vi "Vission Assistant.vi"() -> ()   [LabVIEW 2018]
uses:
  <vilib>/Rock Robotics/Network Tables/NT Read Number.vi
  <vilib>/Rock Robotics/Network Tables/NT Read Boolean.vi
  <vilib>/Rock Robotics/Network Tables/NT Write Number.vi
  <vilib>/Rock Robotics/Network Tables/NT Read Numeric Array.vi
  <vilib>/Rock Robotics/Network Tables/NT Write Boolean.vi
  <vilib>/Rock Robotics/WPI/Utilities/WPI_GetSetVariantRefNum.vi
  <vilib>/Rock Robotics/Network Tables/NT Write Numeric Array.vi
panel:
  out "RobotDrive Motors":dbl[](array[numeric])
  out "Driving Assist Values":dbl[](array[numeric])
  in  "Tab Control":T1(tab)
  in  "High Threshold":dbl=0.9
  in  "Low Threshold":dbl=0.8
  out "Center of Centroid":dbl
  out "Sonar1 Value":dbl
  in  "Wall (Sonar)":dbl=3.0
  in  "Add Left Axis(L)":dbl=0.5499999999999999 min=-1.0 max=1.0 step=0.05
  in  "Add Left Axis(R)":dbl min=-1.0 max=1.0 step=0.05
  in  "Add Right Axis(L)":dbl min=-1.0 max=1.0 step=0.05
  in  "Add Right Axis(R)":dbl=-0.5499999999999999 min=-1.0 max=1.0 step=0.05
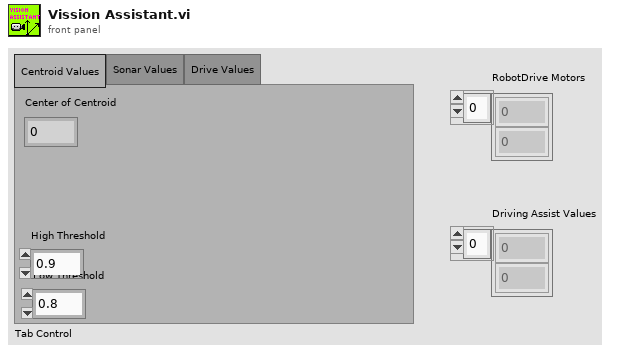
[diagram p1: front panel]
types:
  T1 = enum32{"Centroid Values", "Sonar Values", "Drive Values"}
  T2 = typedef "WPI_RobotDriveDevRef.ctl" = cluster{"DevStatus":errorcluster, "Motors[]":T3[], "Square Inputs":bool, "Max Output":dbl}
  T3 = typedef "WPI_MotorControlDeviceRef.ctl" = cluster{"DeviceStatus":errorcluster, "Type":T4, "PWM":cluster{"PWM Channel":T5, "DeadBand":T6}, "CAN":cluster{"Device Number":u8, "SetOutput VI Ref":variant, "GetOutput VI Ref":variant, "Enable VI Ref":variant, "Disable VI Ref":variant, "Data":variant}, "Invert":bool, "DIO PWM":cluster{"PWM \"Enable\" Channel":T5, "DIOChannel":T7, "PWM Rate":dbl}}
  T4 = typedef "WPI_MotorControlType.ctl" = enum16{"PWM", "CAN", "DIO PWM"}
  T5 = typedef "FPGA_DIOPWMChannel.ctl" = enum8{"PWM 0", "PWM 1", "PWM 2", "PWM 3", "PWM 4", "PWM 5", "PWM 6", "PWM 7", "PWM 8", "PWM 9", "PWM MXP 0", "PWM MXP 1", "PWM MXP 2", "PWM MXP 3", "PWM MXP 4", "PWM MXP 5", "PWM MXP 6", "PWM MXP 7", "PWM MXP 8", "PWM MXP 9", "Invalid"}
  T6 = typedef "WPI_PWMDeadband.ctl" = cluster{"Name":string, "maxPositivePwm":i32, "minPositivePwm":i32, "centerPwm":i32, "maxNegativePwm":i32, "minNegativePwm":i32, "angularRange":u16}
  T7 = typedef "FPGA_DIOChannel.ctl" = enum8{"DIO 0", "DIO 1", "DIO 2", "DIO 3", "DIO 4", "DIO 5", "DIO 6", "DIO 7", "DIO 8", "DIO 9", "DIO MXP 0", "DIO MXP 1", "DIO MXP 2", "DIO MXP 3", "DIO MXP 4", "DIO MXP 5", "DIO MXP 6", "DIO MXP 7", "DIO MXP 8", "DIO MXP 9", "DIO MXP 10", "DIO MXP 11", "DIO MXP 12", "DIO MXP 13", "DIO MXP 14", "DIO MXP 15", "SPI Port CS1", "SPI Port CS2", "SPI Port CS3", "SPI Port MISO", "SPI Port MOSI", "Invalid"}
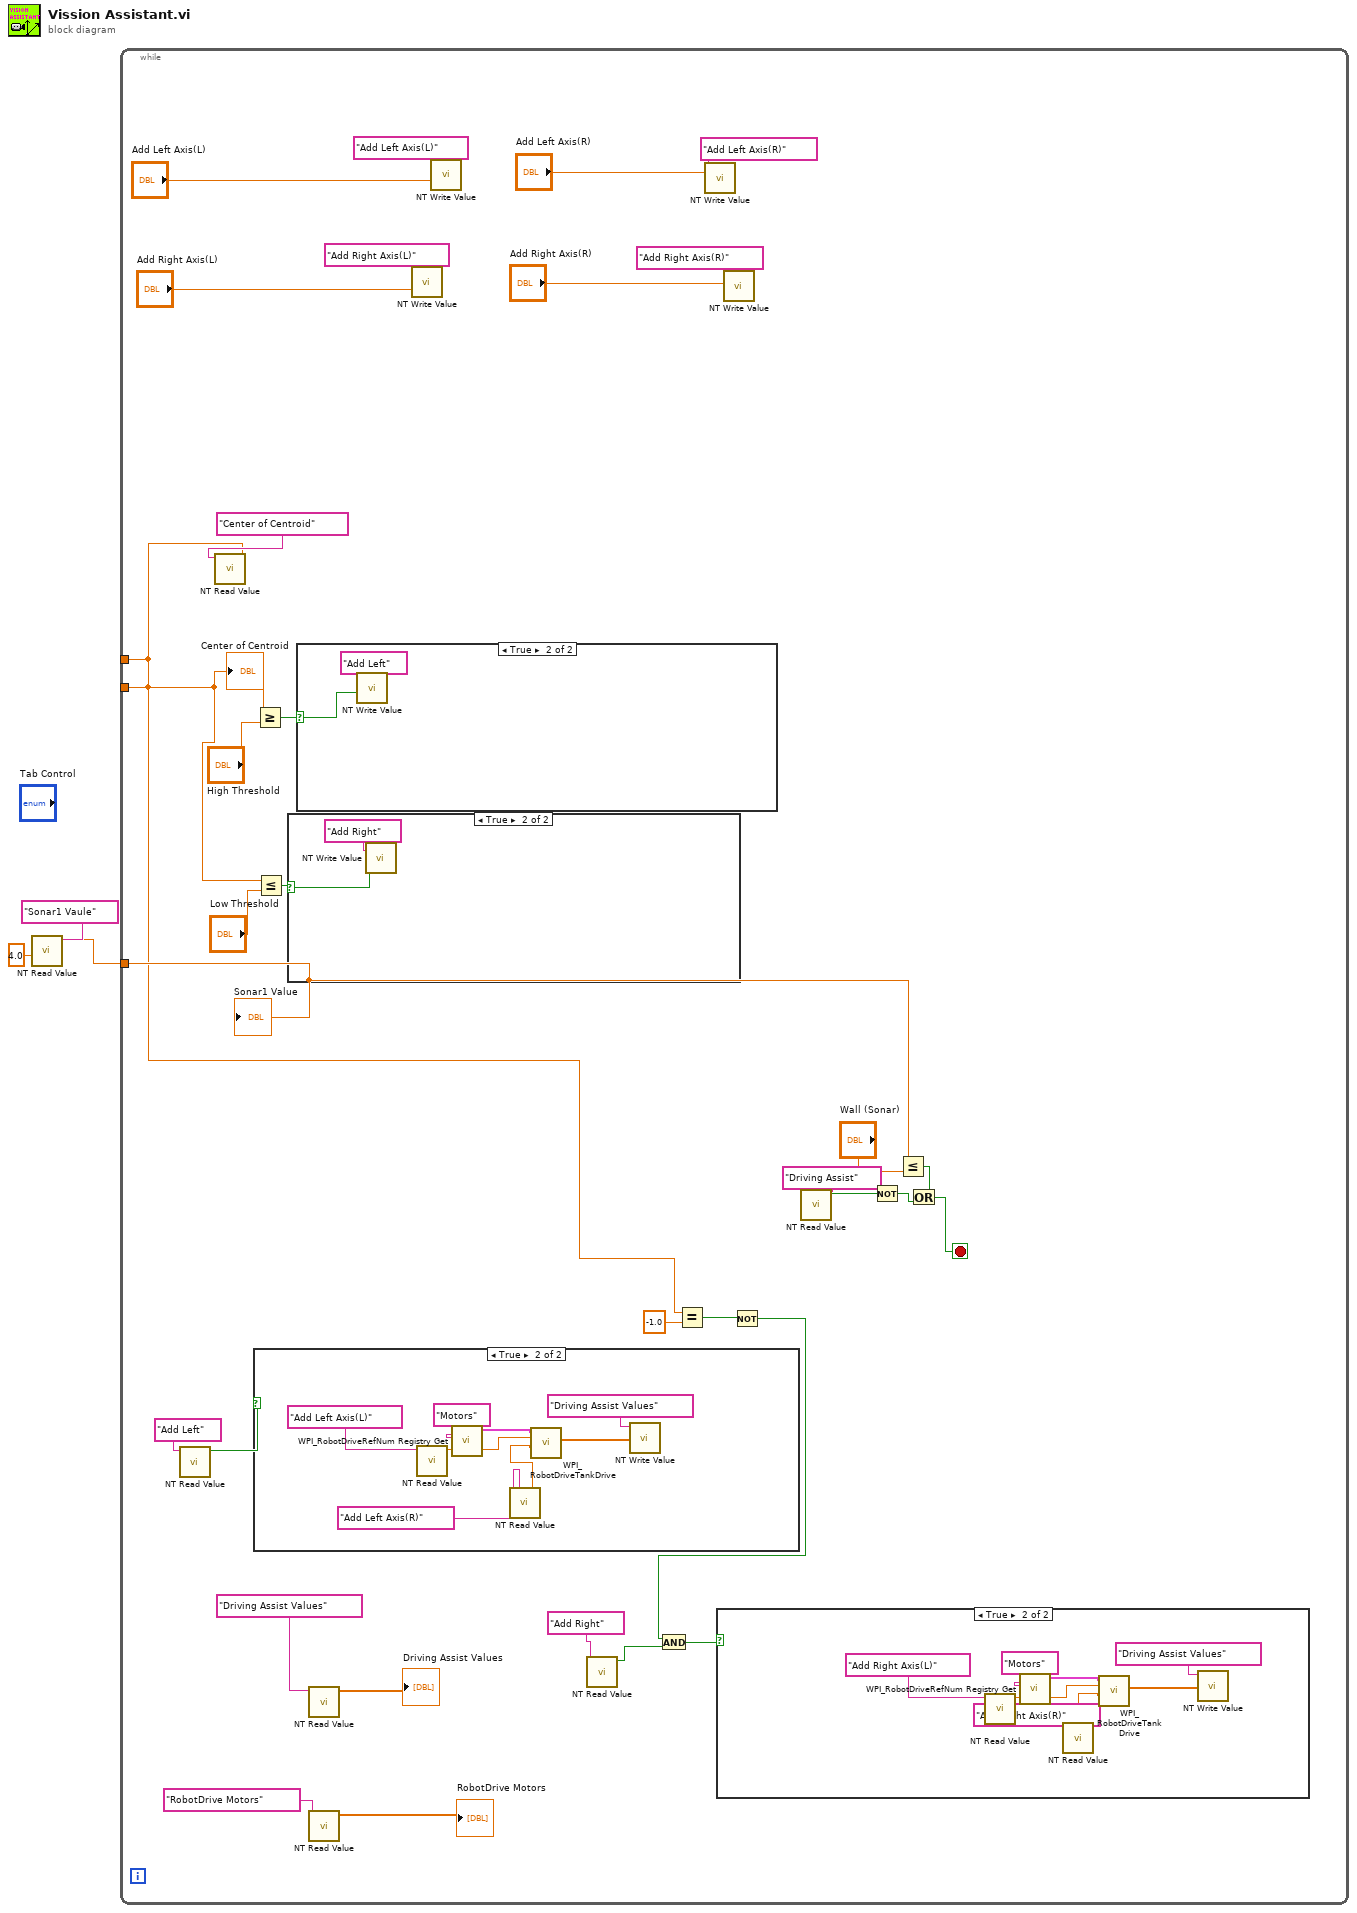
[diagram p0: block diagram]
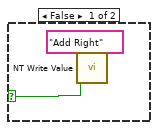
[diagram p4: hidden frame]
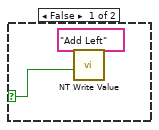
[diagram p5: hidden frame]
diagram:
  n1 = call-poly <vilib>:"NT Read Value.vi"("Default Value"=4.0, "Name"="Sonar1 Vaule") -> ("Numeric"=w2:dbl)  [unwired: 8 in, 1 out]
  n2 = while {
    tunnel: w2 -> [w31]
    tunnel: [w4] -> _
    tunnel: [w4] -> _
    stop <- w14 stop-if-true
    n3 = call-poly <vilib>:"NT Read Value.vi"("Name"="Add Left") -> ("Boolean"=w27:bool)  [unwired: 9 in, 1 out]
    n4 = call-poly <vilib>:"NT Read Value.vi"("Name"="Center of Centroid") -> ("Numeric"=w4:dbl)  [unwired: 9 in, 1 out]
    "Center of Centroid" <- w4
    n5 = case shown="True" w27 {
      frame False {
      }
      frame True {
        n6 = call-poly <vilib>:"NT Read Value.vi"("Name"="Add Left Axis(L)") -> ("Numeric"=w48:dbl)  [unwired: 9 in, 1 out]
        n7 = call <vilib>:"WPI_RobotDriveRefNum Registry Get.vi"("refnum name"="Motors") -> ("RobotDriveDevRef"=w49:T2)  [unwired: 1 in, 9 out]
        n8 = call-poly <vilib>:"NT Read Value.vi"("Name"="Add Left Axis(R)") -> ("Numeric"=w47:dbl)  [unwired: 9 in, 1 out]
        n9 = call <vilib>:"WPI_RobotDriveTankDrive.vi"("Right axis value"=w47, "Left axis value"=w48, "RobotDriveDevRef"=w49) -> ("Motor Values"=w46:dbl[])  [unwired: 6 in, 2 out]
        n10 = call-poly <vilib>:"NT Write Value.vi"("Numeric Array"=w46, "Name"="Driving Assist Values") -> ()  [unwired: 9 in, 1 out]
      }
    }
    n11 = Greater Or Equal?(x=w4, y="High Threshold") -> (x >= y?=w28:bool)
    n12 = Less Or Equal?(x=w4, y="Low Threshold") -> (x <= y?=w29:bool)
    n13 = case shown="True" w29 {
      selector: w29 -> [w53 w56]
      frame False {
        n14 = call-poly <vilib>:"NT Write Value.vi"("Boolean"=w53, "Name"="Add Right") -> ()  [unwired: 9 in, 1 out]
      }
      frame True {
        n15 = call-poly <vilib>:"NT Write Value.vi"("Boolean"=w56, "Name"="Add Right") -> ()  [unwired: 9 in, 1 out]
      }
    }
    n16 = case shown="True" w28 {
      selector: w28 -> [w57 w60]
      frame False {
        n17 = call-poly <vilib>:"NT Write Value.vi"("Boolean"=w57, "Name"="Add Left") -> ()  [unwired: 9 in, 1 out]
      }
      frame True {
        n18 = call-poly <vilib>:"NT Write Value.vi"("Boolean"=w60, "Name"="Add Left") -> ()  [unwired: 9 in, 1 out]
      }
    }
    n19 = call-poly <vilib>:"NT Read Value.vi"("Name"="Driving Assist Values") -> ("Numeric Array"=→"Driving Assist Values":dbl[])  [unwired: 9 in, 1 out]
    n20 = call-poly <vilib>:"NT Read Value.vi"("Name"="RobotDrive Motors") -> ("Numeric Array"=→"RobotDrive Motors":dbl[])  [unwired: 9 in, 1 out]
    n21 = call-poly <vilib>:"NT Write Value.vi"("Numeric"="Add Right Axis(L)", "Name"="Add Right Axis(L)") -> ()  [unwired: 9 in, 1 out]
    n22 = call-poly <vilib>:"NT Write Value.vi"("Numeric"="Add Left Axis(L)", "Name"="Add Left Axis(L)") -> ()  [unwired: 9 in, 1 out]
    n23 = call-poly <vilib>:"NT Read Value.vi"("Name"="Add Right") -> ("Boolean"=w11:bool)  [unwired: 9 in, 1 out]
    n24 = Equal?(x=w4, y=-1.0) -> (x = y?=w10:bool)
    n25 = call-poly <vilib>:"NT Write Value.vi"("Numeric"="Add Left Axis(R)", "Name"="Add Left Axis(R)") -> ()  [unwired: 9 in, 1 out]
    n26 = call-poly <vilib>:"NT Write Value.vi"("Numeric"="Add Right Axis(R)", "Name"="Add Right Axis(R)") -> ()  [unwired: 9 in, 1 out]
    n27 = Not(x=w10) -> (.not. x?=w9:bool)
    n28 = And(x=w9, y=w11) -> (x .and. y?=w12:bool)
    n29 = case shown="True" w12 {
      frame False {
      }
      frame True {
        n30 = call-poly <vilib>:"NT Read Value.vi"("Name"="Add Right Axis(L)") -> ("Numeric"=w40:dbl)  [unwired: 9 in, 1 out]
        n31 = call <vilib>:"WPI_RobotDriveRefNum Registry Get.vi"("refnum name"="Motors") -> ("RobotDriveDevRef"=w41:T2)  [unwired: 1 in, 9 out]
        n32 = call-poly <vilib>:"NT Read Value.vi"("Name"="Add Right Axis(R)") -> ("Numeric"=w39:dbl)  [unwired: 9 in, 1 out]
        n33 = call <vilib>:"WPI_RobotDriveTankDrive.vi"("Right axis value"=w39, "Left axis value"=w40, "RobotDriveDevRef"=w41) -> ("Motor Values"=w38:dbl[])  [unwired: 6 in, 2 out]
        n34 = call-poly <vilib>:"NT Write Value.vi"("Numeric Array"=w38, "Name"="Driving Assist Values") -> ()  [unwired: 9 in, 1 out]
      }
    }
    n35 = call-poly <vilib>:"NT Read Value.vi"("Name"="Driving Assist") -> ("Boolean"=w36:bool)  [unwired: 9 in, 1 out]
    n36 = Not(x=w36) -> (.not. x?=w6:bool)
    n37 = Less Or Equal?(x=w31, y="Wall (Sonar)") -> (x <= y?=w34:bool)
    n38 = Or(x=w34, y=w6) -> (x .or. y?=w14:bool)
    "Sonar1 Value" <- w31
  }
